vi "Perform Action.vi"(8 "error in (no error)":errorcluster, 10 "Input":variant, 11 "DIO DAQmx PWM CFG in":refnum<class "CO DAQmx PWM CFG.lvclass">) -> (0 "error out":errorcluster, 2 "Output":variant, 3 "DIO DAQmx PWM CFG out":refnum<class "CO DAQmx PWM CFG.lvclass">)   [LabVIEW 2024, in "CO DAQmx PWM CFG.lvclass"]
uses:
  CO DAQmx PWM CFG.lvclass
  DAQmx Base CFG/DAQmx Base CFG.lvclass/DAQmx Base CFG.ctl
  DAQmx Base CFG/DAQmx Base CFG.lvclass
  <resource>/objmgr/daqmx.rc
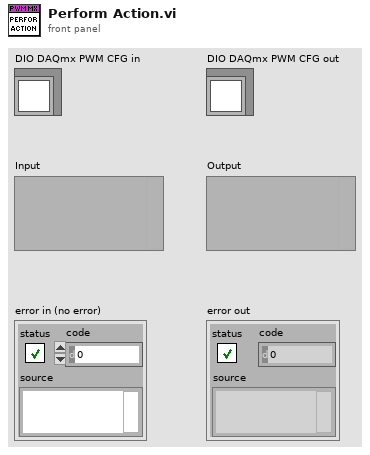
[diagram p1: front panel]
types:
  T1 = cluster{"Channel":string, "PWM Pams":cluster{"Frequency":dbl, "Duty Cycle":dbl}}
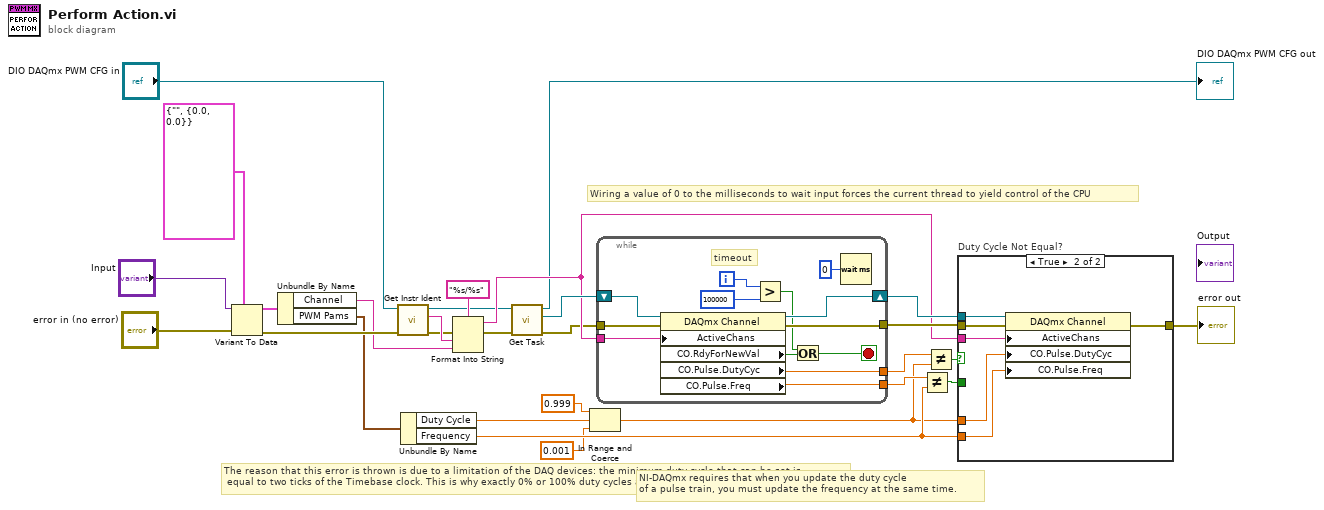
[diagram p0: block diagram]
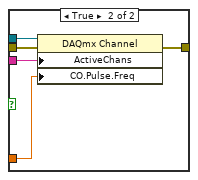
[diagram p3: hidden frame]
diagram:
  # "The reason that this error is thrown is due to a limitation of the DAQ devices: the minimum duty cycle that can be set is\n equal to two ticks of the Timebase clock. This is why exactly 0% or 100% duty cycles are not possible."
  # "Wiring a value of 0 to the milliseconds to wait input forces the current thread to yield control of the CPU"
  # "NI-DAQmx requires that when you update the duty cycle\nof a pulse train, you must update the frequency at the same time."
  n1 = Variant To Data(error in="error in (no error)", type=T1 {"Channel"="", "PWM Pams"={"Frequency"=0.0, "Duty Cycle"=0.0}}, Variant="Input") -> (data=w24:T1, error out=w25:errorcluster)
  n2 = Unbundle By Name(w24) -> ("Channel"=w19:string, "PWM Pams"=w17:cluster{"Frequency":dbl, "Duty Cycle":dbl})
  n3 = call-dynamic "Get Instr Ident.vi"("error in"=w25, "CFG JSON in"="DIO DAQmx PWM CFG in") -> ("error out"=w18:errorcluster, "Instr Ident"=w20:string, "CFG JSON out"=w6:refnum<class "CO DAQmx PWM CFG.lvclass">)  [unwired: 7 in]
  n4 = Unbundle By Name(w17) -> ("Duty Cycle"=w15:dbl, "Frequency"=w11:dbl)
  n5 = Format Into String(format string="%s/%s", error in=w18, w20, w19) -> (resulting string=w7:string, error out=w2:errorcluster)  [unwired: 1 in]
  n6 = call "Get Task.vi"("DAQmx Base CFG in"=w6) -> ("Task"=w10:refnum<k21>, "DAQmx Base CFG out"=→"DIO DAQmx PWM CFG out":refnum<class "CO DAQmx PWM CFG.lvclass">)  [unwired: 9 in]
  n7 = In Range and Coerce(upper limit=0.999, x=w15, lower limit=0.001) -> (coerced(x)=w5:dbl)  [unwired: 1 out]
  n8 = while {
    tunnel: [w40] -> w14
    tunnel: w2 -> [w39]
    tunnel: [w37] -> w9
    tunnel: w7 -> [w36]
    shift-right: [w41] -> w16
    shift-left: w10 -> [w38]
    tunnel: [w30] -> w8
    i -> [w34]
    stop <- w32 stop-if-true
    # "timeout"
    n9 = property class="DAQmx Channel"(reference=w38, error in=w39, "ActiveChans"=w36) -> (reference out=w41:refnum<k21>, error out=w30:errorcluster, "CO.RdyForNewVal"=w35:bool, "CO.Pulse.DutyCyc"=w40:dbl, "CO.Pulse.Freq"=w37:dbl)
    n10 = Greater?(x=w34, y=100000) -> (0:w29:bool)
    n11 = Or(x=w29, y=w35) -> (x .or. y?=w32:bool)
    n12 = Wait (ms)(milliseconds to wait=u32 0) -> ()  [unwired: 1 out]
  }
  n13 = Not Equal?(x=w9, y=w11) -> (x != y?=w12:bool)
  n14 = Not Equal?(x=w14, y=w5) -> (x != y?=w13:bool)
  n15 = case "Duty Cycle Not Equal?" shown="True" w13 {
    tunnel: [w44 w59] -> w22
    tunnel: w11 -> [w45 w58]
    tunnel: w8 -> [w47 w57]
    tunnel: w16 -> [w43 w56]
    tunnel: w5 -> [_ w55]
    tunnel: w12 -> [w46 _]
    tunnel: w7 -> [w42 w54]
    frame False {
      n16 = case "Frequeny Not Equal?" shown="False" w46 {
        tunnel: w47 -> [w48 w53]
        tunnel: w45 -> [_ w50]
        tunnel: [w48 w52] -> w44
        tunnel: w43 -> [_ w51]
        tunnel: w42 -> [_ w49]
        frame False {
        }
        frame True {
          n17 = property class="DAQmx Channel"(reference=w51, error in=w53, "ActiveChans"=w49, "CO.Pulse.Freq"=w50) -> (error out=w52:errorcluster)  [unwired: 1 out]
        }
      }
    }
    frame True {
      n18 = property class="DAQmx Channel"(reference=w56, error in=w57, "ActiveChans"=w54, "CO.Pulse.DutyCyc"=w55, "CO.Pulse.Freq"=w58) -> (error out=w59:errorcluster)  [unwired: 1 out]
    }
  }
  "error out" <- w22
